vi "Read Scanner Data.vi"(8 "error in (no error)":errorcluster, 11 "Scannable in":refnum<class "Scannable.lvclass">) -> (0 "error out":errorcluster, 3 "Scannable out":refnum<class "Scannable.lvclass">)   [LabVIEW 2009, in "Scannable.lvclass"]
uses:
  Scannable.lvclass
panel:
  out "Channel Names":string[](array[string])
  out "Channel Units":string[](array[string])
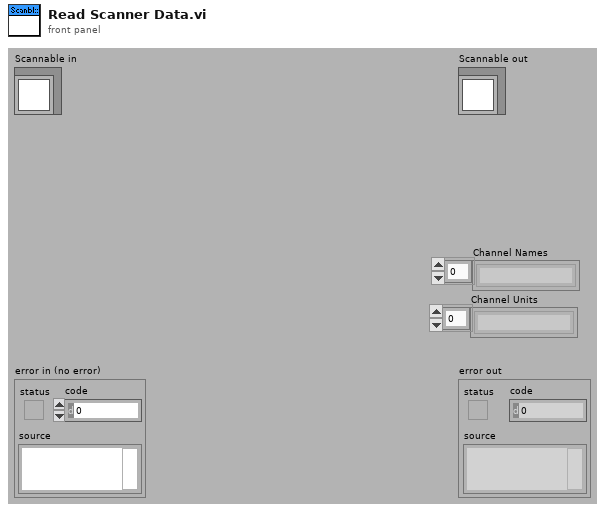
[diagram p1: front panel]
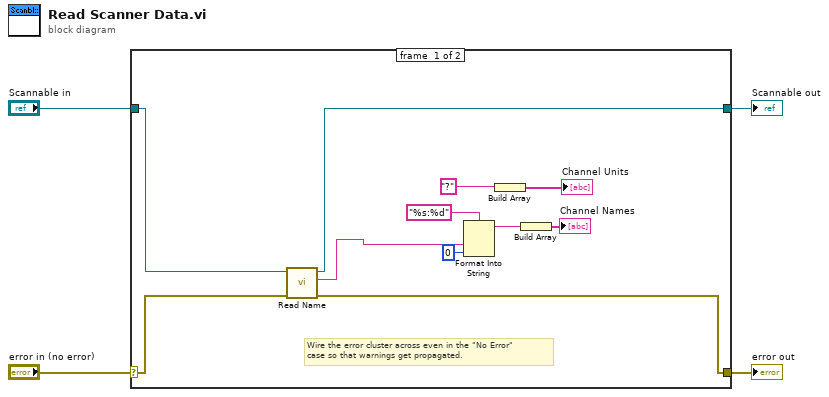
[diagram p0: block diagram]
diagram:
  n1 = case shown="No Error" "error in (no error)" {
    selector: "error in (no error)" -> [w11 w17]
    tunnel: [w10 w17] -> w3
    tunnel: [w9 w16] -> w1
    tunnel: "Scannable in" -> [w12 w16]
    frame #0 {
      # "Wire the error cluster across even in the \"No Error\"\ncase so that warnings get propagated."
      n2 = call-dynamic "Read Name.vi"("error in (no error)"=w11, "Instrument.lvclass in"=w12) -> ("error out"=w10:errorcluster, "Name"=w15:string, "Instrument.lvclass out"=w9:refnum<class "Scannable.lvclass">)  [unwired: 7 out]
      n3 = Format Into String(format string="%s:%d", w15, 0 ("input 2")) -> (resulting string=w14:string)  [unwired: 2 in, 1 out]
      n4 = Build Array("?" ("resulting string")) -> (→"Channel Units":string[])
      n5 = Build Array(w14) -> (→"Channel Names":string[])
    }
    frame #1 {
    }
  }
  "error out" <- w3
  "Scannable out" <- w1
